vi "FTW-Container-Type.vi"(0 "FTW-Container In":refnum<class "FTW-Container.lvclass">, 11 "error in":errorcluster) -> (4 "FTW-Container Out":refnum<class "FTW-Container.lvclass">, 8 "Type":T1, 15 "error out":errorcluster)   [LabVIEW 2015, in "FTW-Container.lvclass"]
uses:
  FTW-Container.lvclass
  <vilib>/Utility/Data Type/Type Definitions/Data Type.ctl
  FTW-Container.lvclass/FTW-Container.ctl
  <vilib>/Utility/Data Type/NI_Data Type.lvlib
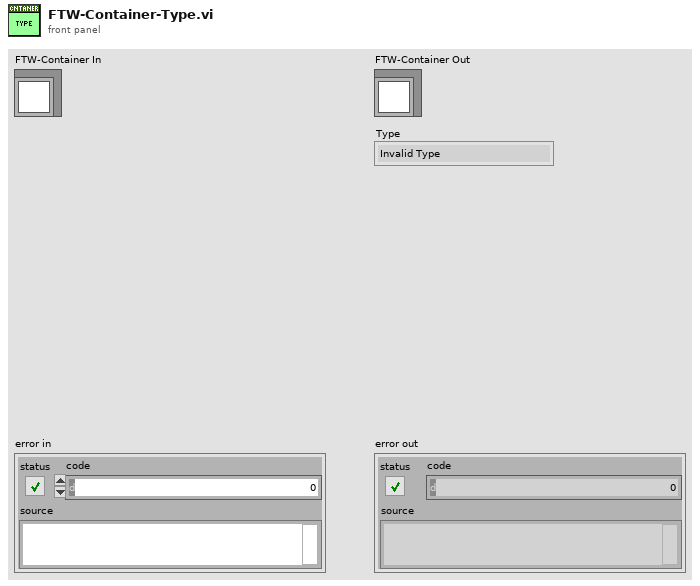
[diagram p1: front panel]
types:
  T1 = typedef "NI_Data Type.lvlib/Data Type.ctl" = enum8{"Invalid Type", "Void", "I8", "I16", "I32", "I64", "U8", "U16", "U32", "U64", "Single Float", "Double Float", "Extended Float", "Single Complex", "Double Complex", "Extended Complex", "Enum U8", "Enum U16", "Enum U32", "Enum U64", "Single Float With Unit", "Double Float With Unit", "Extended Float With Unit", "Single Complex with Unit", "Double Complex with Unit", "Extended Complex with Unit", "Boolean", "String", "Path", "Picture", "Tag", "Array", "Cluster", "Variant", "LV Variant", "Waveform", "Timestamp", "Digital Waveform", "Digital Data", "ExpressData", "Refnum", "External Data", "VI", "Poly VI", "LabVIEW Class Instance", "Fixed Point"}
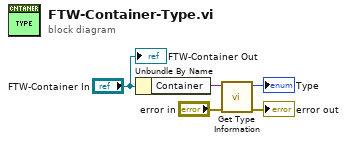
[diagram p0: block diagram]
diagram:
  n1 = Unbundle By Name("FTW-Container In") -> ("Container"=w1:variant)
  n2 = call <vilib>:"Get Type Information.vi"("error in (no error)"="error in", "Variant"=w1) -> ("error out"=→"error out":errorcluster, "Type"=→"Type":T1)  [unwired: 5 in, 3 out]
  "FTW-Container Out" <- "FTW-Container In"
